vi "File_ListDirectoryRecursivly.vi"(0 "DirPath":path, 1 "Treat LLB as directories?":bool, 2 "Delete cache before?":bool=TRUE, 5 "error in (no error)":errorcluster) -> (15 "Files":path[](array[path]), 19 "error out":errorcluster)   [LabVIEW 2014]
doc: "Lists a directory recursively."
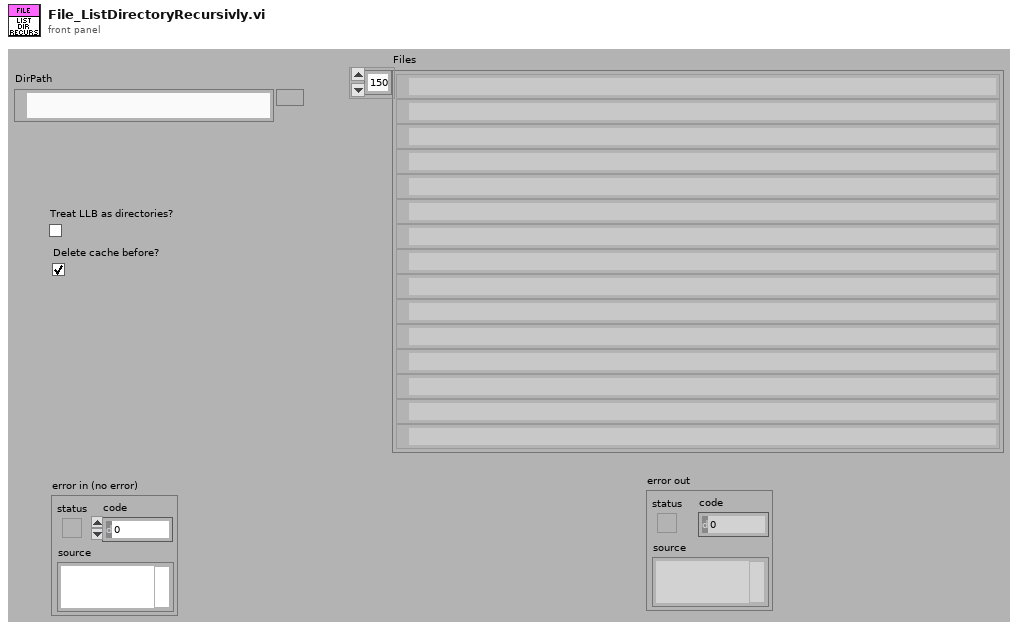
[diagram p1: front panel]
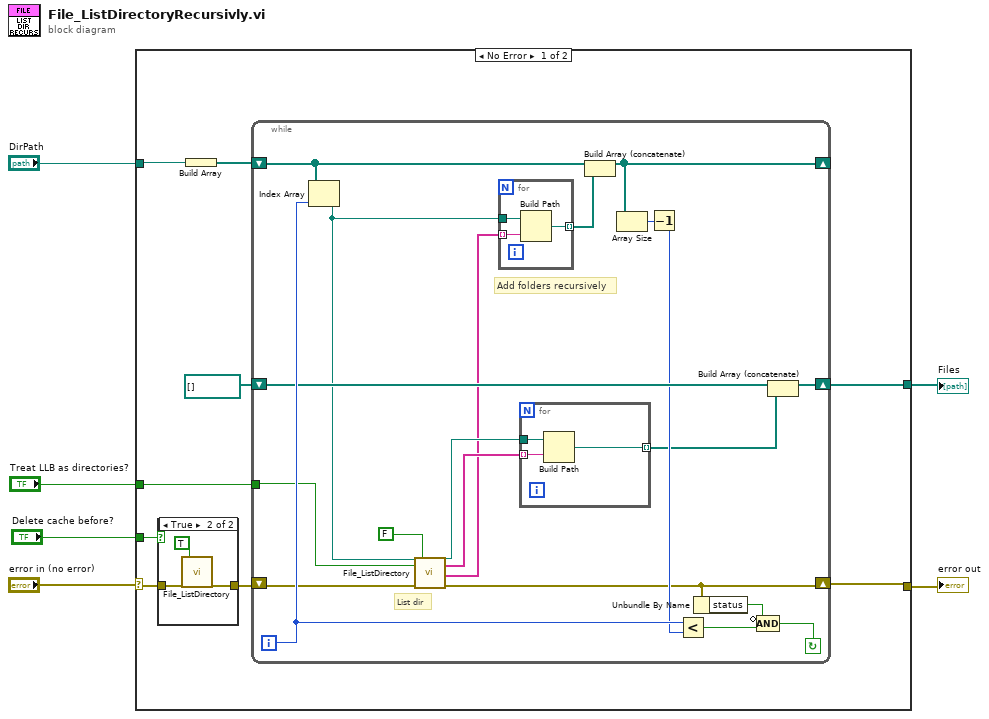
[diagram p0: block diagram]
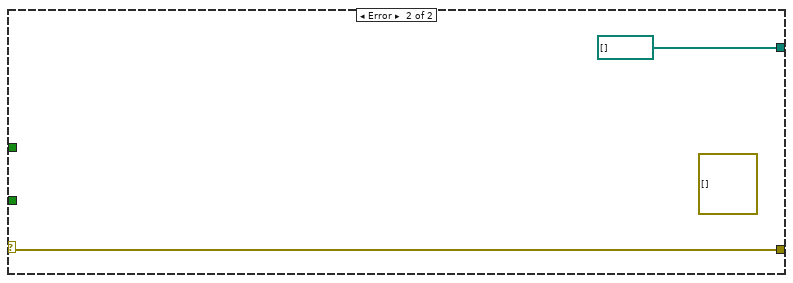
[diagram p3: hidden frame]
diagram:
  n1 = case shown="No Error" "error in (no error)" {
    selector: "error in (no error)" -> [w10 w47]
    tunnel: [w14 w47] -> w5
    tunnel: "DirPath" -> [w8 _]
    tunnel: "Treat LLB as directories?" -> [w13 _]
    tunnel: [w12 path[] [] ("Files")] -> w2
    tunnel: "Delete cache before?" -> [w7 _]
    frame No Error {
      n2 = case shown="True" w7 {
        tunnel: w10 -> [w42 w45]
        tunnel: [w42 w44] -> w9
        frame False {
        }
        frame True {
          n3 = call <resource>:"File_ListDirectory.vi"("error in (no error)"=w45, "Reset"=TRUE) -> ("error out"=w44:errorcluster)  [unwired: 3 in, 14 out]
        }
      }
      n4 = Build Array(w8) -> (w15:path[])
      n5 = while {
        shift-left: path[] [] ("Files") -> [w26]
        shift-right: [w27] -> w12
        tunnel: w13 -> [w23]
        shift-left: w15 -> [w34]
        shift-right: [w33] -> _
        shift-left: w9 -> [w25]
        shift-right: [w16] -> w14
        i -> [w31]
        stop <- w28 continue-if-true
        # "Add folders recursively"
        # "List dir"
        n6 = Index Array(array=w34, index=w31) -> (element=w24:path)
        n7 = call <resource>:"File_ListDirectory.vi"("Directory Path"=w24, "Treat LLB as directories?"=w23, "error in (no error)"=w25, "Reset"=FALSE) -> ("Dup directory path"=w20:path, "File names"=w19:string[], "Directory names"=w17:string[], "error out"=w16:errorcluster)  [unwired: 1 in, 11 out]
        n8 = for {
          tunnel: w17 -> [w41] mode=indexing
          tunnel: w24 -> [w40]
          tunnel: [w39] -> w35 mode=indexing
          n9 = Build Path(base path=w40, name or relative path=w41) -> (appended path=w39:path)
        }
        n10 = for {
          tunnel: w20 -> [w38]
          tunnel: w19 -> [w37] mode=indexing
          tunnel: [w36] -> w18 mode=indexing
          n11 = Build Path(base path=w38, name or relative path=w37) -> (appended path=w36:path)
        }
        n12 = Build Array (concatenate)(w34, w35) -> (w33:path[])
        n13 = Array Size(array=w33) -> (size(s)=w32:i32)
        n14 = Decrement(x=w32) -> (x-1=w21:i32)
        n15 = Less?(x=w31, y=w21) -> (x < y?=w30:bool)
        n16 = Unbundle By Name(w16) -> ("status"=w29:bool)
        n17 = Compound Arithmetic op=AND(invert w29, w30) -> (w28:bool)
        n18 = Build Array (concatenate)(w26, w18) -> (w27:path[])
      }
    }
    frame Error {
      (unwired) errorcluster[] []
    }
  }
  "error out" <- w5
  "Files" <- w2
